vi "Funcion_Cierre_B.vi"(9 "PIPES":cluster{"PIPE_IN":i32, "PIPE_OUT":i32}, 11 "error in (no error)":errorcluster) -> (2 "Cierre":bool, 3 "error out":errorcluster)   [LabVIEW 2016]
uses:
  microchip_solutions_v2013-06-15/USB/Tools/MCHPUSB Custom Driver/Mpusbapi/Dll/Borland_C/mpusbapi.dll
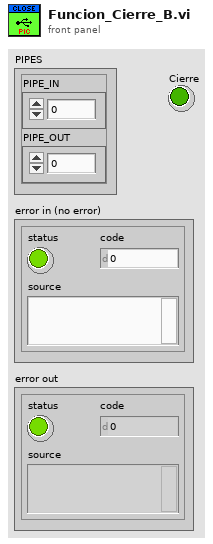
[diagram p1: front panel]
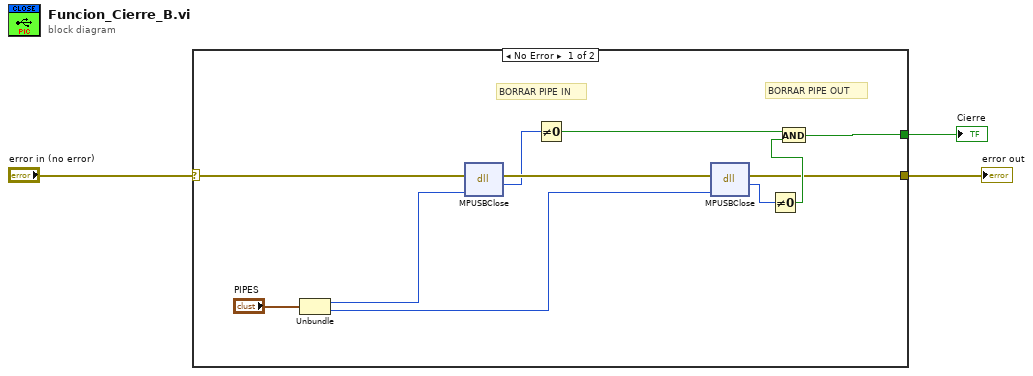
[diagram p0: block diagram]
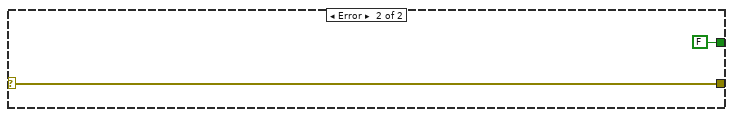
[diagram p2: hidden frame]
diagram:
  n1 = case shown="No Error" "error in (no error)" {
    selector: "error in (no error)" -> [w6 w16]
    tunnel: [w5 w16] -> w2
    tunnel: [w4 FALSE] -> w1
    frame No Error {
      # "BORRAR PIPE OUT"
      # "BORRAR PIPE IN"
      n2 = Unbundle("PIPES") -> ("PIPE_IN"=w12:i32, "PIPE_OUT"=w13:i32)
      n3 = dll-call lib="C:/microchip_solutions_v2013-06-15/USB/Tools/MCHPUSB Custom Driver/Mpusbapi/Dll/Borland_C/mpusbapi.dll" fn="MPUSBClose"(error in=w6, "HANDLE"=w12) -> (error out=w11:errorcluster, "CIERRE"=w9:i32)  [unwired: 3 in, 1 out]
      n4 = Not Equal To 0?(x=w9) -> (x != 0?=w10:bool)
      n5 = dll-call lib="C:/microchip_solutions_v2013-06-15/USB/Tools/MCHPUSB Custom Driver/Mpusbapi/Dll/Borland_C/mpusbapi.dll" fn="MPUSBClose"(error in=w11, "HANDLE"=w13) -> (error out=w5:errorcluster, "CIERRE"=w8:i32)  [unwired: 3 in, 1 out]
      n6 = Not Equal To 0?(x=w8) -> (x != 0?=w7:bool)
      n7 = And(x=w10, y=w7) -> (x .and. y?=w4:bool)
    }
    frame Error {
    }
  }
  "error out" <- w2
  "Cierre" <- w1
